vi "VI_Execution_State.vi"(8 "error in (no error)":errorcluster, 11 "UI_Interaction_Manager in":refnum<class "UI_Interaction_Manager.lvclass">) -> (0 "error out":errorcluster, 1 "Running?":bool, 2 "Execution:State":T1(ring), 3 "UI_Interaction_Manager out":refnum<class "UI_Interaction_Manager.lvclass">)   [LabVIEW 2011, in "UI_Interaction_Manager.lvclass"]
uses:
  UI_Interaction_Manager.lvclass
  UI_Interaction_Manager.lvclass/UI_Interaction_Manager.ctl
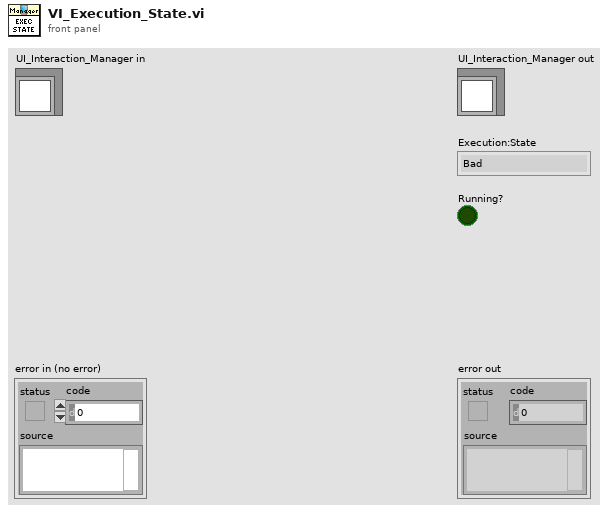
[diagram p1: front panel]
types:
  T1 = enum32{"Bad", "Idle", "Run top level", "Running"}
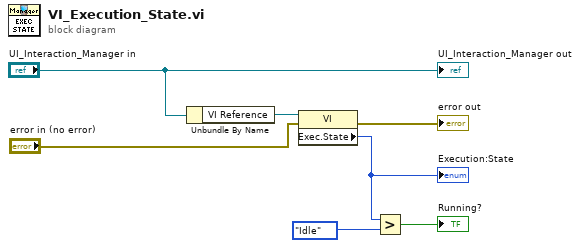
[diagram p0: block diagram]
diagram:
  n1 = Unbundle By Name("UI_Interaction_Manager in") -> ("VI Reference"=w4:refnum<vi>)
  n2 = property class="VI"(reference=w4, error in="error in (no error)") -> (error out=→"error out":errorcluster, "Exec.State"=w2:T1)  [unwired: 1 out]
  "Execution:State" <- w2
  n3 = Greater?(x=w2, y=T1."Idle") -> (0:→"Running?":bool)
  "UI_Interaction_Manager out" <- "UI_Interaction_Manager in"
